vi "Load Memory Types.vi"(8 "error in (no error)":errorcluster, 11 "Sequencing in":refnum<class "Sequencing.lvclass">) -> (0 "error out":errorcluster, 3 "Sequencing out":refnum<class "Sequencing.lvclass">)   [LabVIEW 2020, in "VolatusSeq.lvlib" / "Sequencing.lvclass"]
uses:
  Sequencing.lvclass
  Sequencing.lvclass/Sequencing.ctl
  VolatusSeq.lvlib
  VolatusSeqConfig/Condition Config/Condition Config.lvclass
  VolatusSeqConfig/Transition Config/Transition Config.lvclass
  VolatusSeqConfig/VolatusSeqConfig.lvlib
  VolatusSeqConfig/Command Type.ctl
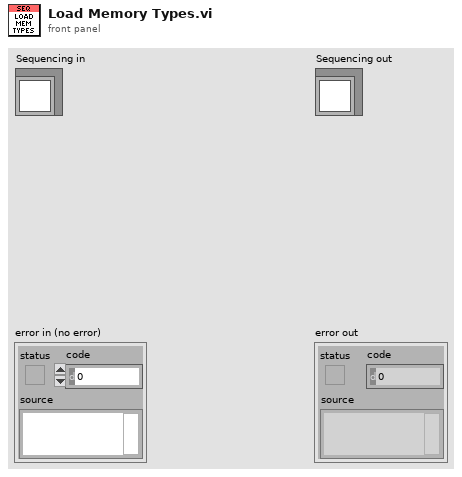
[diagram p1: front panel]
types:
  T1 = typedef "VolatusSeqConfig.lvlib/Command Type.ctl" = enum16{"Digital", "Numeric", "Transition", "Stop", "StartLog", "StopLog", "Start", "Event", "Error", "HTTP", "ResetVar", "IncVar", "DecVar", "SaveVar", "LoadVar", "AddVar", "SubVar", "SetVar"}
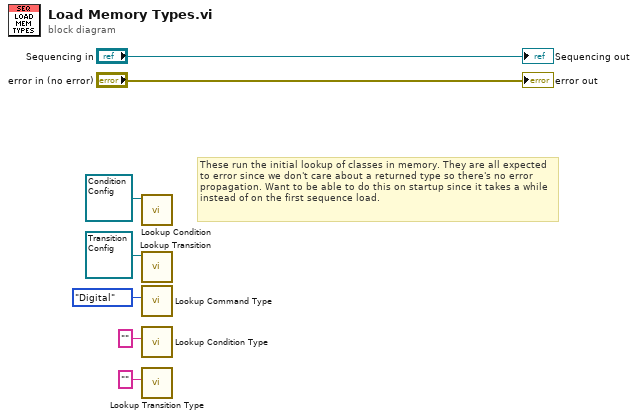
[diagram p0: block diagram]
diagram:
  # "These run the initial lookup of classes in memory. They are all expected to error since we don't care about a returned type so there's no error propagation. Want to be able to do this on startup since it takes a while instead of on the first sequence load."
  n1 = call "Lookup Condition.vi"("Condition Config"=refnum<class "Condition Config.lvclass"> refnum) -> ()  [unwired: 9 in, 2 out]
  n2 = call "Lookup Transition.vi"("Transition Config"=refnum<class "Transition Config.lvclass"> refnum) -> ()  [unwired: 9 in, 2 out]
  n3 = call "Lookup Command Type.vi"("Command Type"=Command_Type."Digital") -> ()  [unwired: 9 in, 2 out]
  n4 = call "Lookup Condition Type.vi"("Condition Type"="") -> ()  [unwired: 9 in, 2 out]
  n5 = call "Lookup Transition Type.vi"("Transition Type"="") -> ()  [unwired: 9 in, 2 out]
  "error out" <- "error in (no error)"
  "Sequencing out" <- "Sequencing in"
